vi "PH_Cont-601k_PowerUnit.set safe state.vi"(0 "i ref in":refnum<vi>, 5 "error in (no error)":errorcluster) -> (14 "i ref out":refnum<vi>, 19 "error out":errorcluster)   [LabVIEW 2014, in "PH_Cont-601k_PowerUnit.lvlib"]
doc: "This VI set \"inistate SM\", set GUI element \"PU on\" = false, unregister PSU Info Tags, set GUI elements \"PSU Info\" = 0, set attribute \"PU on\" = false"
uses:
  PH_Cont-601k_PowerUnit.lvlib
  PH_Devices/PH_Cont-601k_PSU/PH_Cont-601k_PSU.Mode.ctl
  PH_Devices/PH_Cont-601k_PSU/PH_Cont-601k_PSU.Configuration.ctl
  PH_Devices/PH_Cont-601k_PSU/PH_Cont-601k_PSU.lvlib
  PH_Basics/PH_PowerUnit_BaseClass/PH_PowerUnit_BaseClass.lvlib
  CS_Core/BaseSM/BaseSM.lvlib
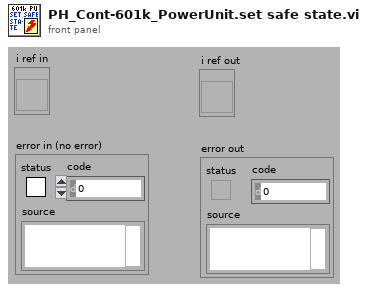
[diagram p1: front panel]
types:
  T1 = typedef "PH_Cont-601k_PSU.lvlib/PH_Cont-601k_PSU.Mode.ctl" = enum32{"STOP", "STANDBY", "READY", "EMISSION", "ERROR"}
  T2 = typedef "PH_Cont-601k_PSU.lvlib/PH_Cont-601k_PSU.Configuration.ctl" = u16
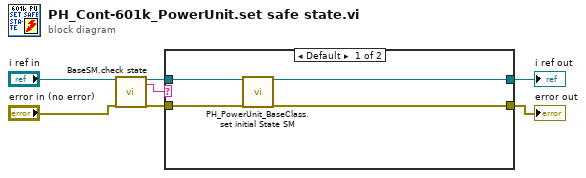
[diagram p0: block diagram]
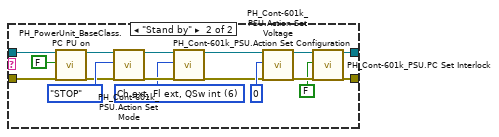
[diagram p2: hidden frame]
diagram:
  n1 = call "BaseSM.check state.vi"("i ref in"="i ref in", "error in (no error)"="error in (no error)") -> ("i ref out"=w2:refnum<vi>, "actualState"=w1:string, "error out"=w4:errorcluster)  [unwired: 12 in, 3 out]
  n2 = case shown="Default" w1 {
    tunnel: [w10 w15] -> w7
    tunnel: [w9 w14] -> w6
    tunnel: w4 -> [w11 w13]
    tunnel: w2 -> [w8 w12]
    frame Default {
      n3 = call "PH_PowerUnit_BaseClass.set initial State SM.vi"("VI in"=w8, "error in (no error)"=w11) -> ("VI out"=w10:refnum<vi>, "error out"=w9:errorcluster)  [unwired: 16 in]
    }
    frame "Stand by" {
      w19 = T2 6 items=["Ch intl, Fl intl, QSw intl", "Ch intl, Fl intl, QSw ext", "Ch intl, Fl ext, QSw intl", "Ch intl, Fl ext, QSw ext", "Ch ext, Fl int, QSw int", "Ch ext, Fl int, QSw ext", "Ch ext, Fl ext, QSw int", "Ch ext, Fl ext, QSw ext"] ("Configuration")
      n4 = call "PH_PowerUnit_BaseClass.PC PU on.vi"("i ref in"=w12, "PU on"=FALSE, "error in (no error)"=w13) -> ("i ref out"=w17:refnum<vi>, "error out"=w18:errorcluster)  [unwired: 15 in]
      n5 = call "PH_Cont-601k_PSU.Action Set Mode.vi"("VI in"=w17, "Mode"=PH_Cont-601k_PSU.Mode."STOP" ("Mode to set"), "error in (no error)"=w18) -> ("VI out"=w21:refnum<vi>, "error out"=w28:errorcluster)  [unwired: 15 in]
      n6 = call "PH_Cont-601k_PSU.Action Set Configuration.vi"("VI in"=w21, "Configuration"=w19, "error in (no error)"=w28) -> ("VI out"=w20:refnum<vi>, "error out"=w22:errorcluster)  [unwired: 15 in]
      n7 = call "PH_Cont-601k_PSU.Action Set Voltage.vi"("VI in"=w20, "Voltage [V]"=u16 0, "error in (no error)"=w22) -> ("VI out"=w27:refnum<vi>, "error out"=w26:errorcluster)  [unwired: 15 in]
      n8 = call "PH_Cont-601k_PSU.PC Set Interlock.vi"("VI in"=w27, "Set Interlock"=FALSE, "error in (no error)"=w26) -> ("VI out"=w15:refnum<vi>, "error out"=w14:errorcluster)  [unwired: 15 in]
    }
  }
  "error out" <- w6
  "i ref out" <- w7
